vi "Switch Close Test.vi"(6 "Driver Refs":T2, 8 "error in (no error)":errorcluster, 11 "SWI Instrument Record":T1) -> (0 "error out":errorcluster {"code" format="%.0x"})   [LabVIEW 2011]
uses:
  TypeDefs/Switch Driver Refs.ctl
  drivers/SWI/SWI Driver Ref.ctl
  drivers/PFE/PFE Driver Ref.ctl
  server/database/Stations/Instruments/Instrument Record.ctl
  drivers/SWI/SWI Command.ctl
  drivers/PFE/PFE Command.ctl
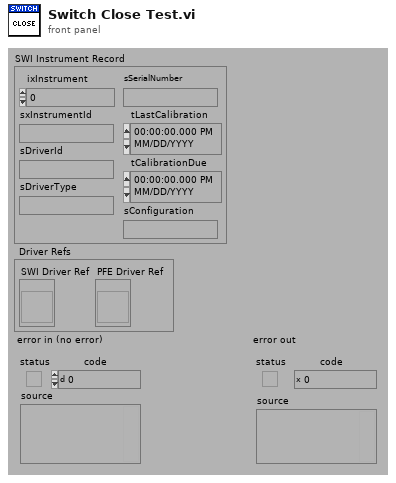
[diagram p1: front panel]
types:
  T1 = typedef "Instrument Record.ctl" = cluster{"ixInstrument":i32, "sxInstrumentId":string, "sDriverId":string, "sDriverType":string, "sSerialNumber":string, "tLastCalibration":timestamp, "tCalibrationDue":timestamp, "sConfiguration":string}
  T2 = typedef "Switch Driver Refs.ctl" = cluster{"SWI Driver Ref":T3, "PFE Driver Ref":T4}
  T3 = typedef "SWI Driver Ref.ctl" = refnum<vi>
  T4 = typedef "PFE Driver Ref.ctl" = refnum<vi>
  T5 = typedef "SWI Command.ctl" = enum16{"LOAD", "INITIALIZE", "PRESET", "SET STIMULUS", "GET STIMULUS", "GET INFO", "RELEASE", "UNLOAD"}
  T6 = typedef "PFE Command.ctl" = enum16{"LOAD", "INITIALIZE", "PRESET", "SET STIMULUS", "GET STIMULUS", "GET INFO", "RELEASE", "UNLOAD"}
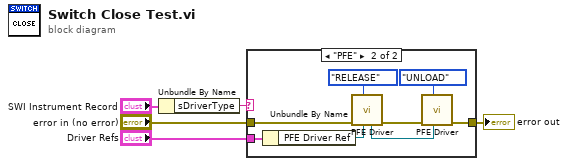
[diagram p0: block diagram]
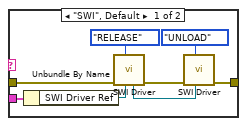
[diagram p2: hidden frame]
diagram:
  n1 = Unbundle By Name("SWI Instrument Record") -> ("sDriverType"=w1:string)
  n2 = case shown="\"PFE\"" w1 {
    tunnel: [w9 w17] -> w5
    tunnel: "Driver Refs" -> [w7 w15]
    tunnel: "error in (no error)" -> [w8 w16]
    frame "SWI", Default {
      n3 = Unbundle By Name(w7) -> ("SWI Driver Ref"=w6:T3)
      n4 = call "SWI Driver.vi"("Drv Refnum"=w6, "SWI Command"=SWI_Command."RELEASE", "error in (no error)"=w8) -> ("error out"=w11:errorcluster, "dup Drv Refnum"=w10:T3)  [unwired: 2 in, 5 out]
      n5 = call "SWI Driver.vi"("Drv Refnum"=w10, "SWI Command"=SWI_Command."UNLOAD", "error in (no error)"=w11) -> ("error out"=w9:errorcluster)  [unwired: 2 in, 6 out]
    }
    frame "PFE" {
      n6 = Unbundle By Name(w15) -> ("PFE Driver Ref"=w14:T4)
      n7 = call "PFE Driver.vi"("Drv Refnum"=w14, "PFE Command"=PFE_Command."RELEASE", "error in (no error)"=w16) -> ("error out"=w19:errorcluster, "dup Drv Refnum"=w18:T4)  [unwired: 5 in, 2 out]
      n8 = call "PFE Driver.vi"("Drv Refnum"=w18, "PFE Command"=PFE_Command."UNLOAD", "error in (no error)"=w19) -> ("error out"=w17:errorcluster)  [unwired: 5 in, 3 out]
    }
  }
  "error out" <- w5
